vi "SetPoint.vi"(8 "error in (no error)":errorcluster, 10 "Point":cluster{"x":i16, "y":i16}, 11 "Point in":refnum<class "Point.lvclass">) -> (0 "error out":errorcluster, 3 "Point out":refnum<class "Point.lvclass">)   [LabVIEW 2021, in "Picture2D.lvlib" / "Point.lvclass"]
uses:
  Point.lvclass
  Point.lvclass/Point.ctl
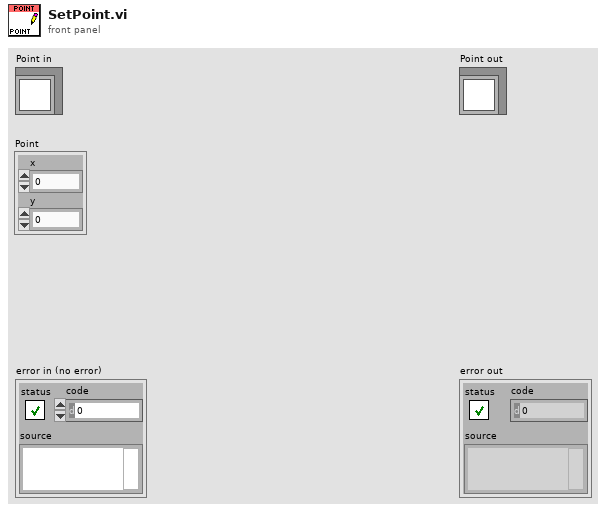
[diagram p1: front panel]
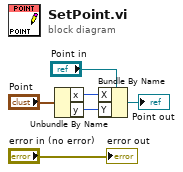
[diagram p0: block diagram]
diagram:
  n1 = Unbundle By Name("Point") -> ("x"=w3:i16, "y"=w2:i16)
  n2 = Bundle By Name(cluster="Point in", "X"=w3, "Y"=w2) -> (→"Point out":refnum<class "Point.lvclass">)
  "error out" <- "error in (no error)"
